vi "PanelPrincipal.vi"() -> ()   [LabVIEW 2020]
panel:
  out "Waveform Chart":dynamicdata(graph)
  out "V2":bool
  out "Motor2":bool
  out "Motor1":bool
  out "V1":bool
  in  "stop":bool caption="Parada"
  out "Multi-Segment Pipe 7":bool(c317)
  out "Tanque 2":dbl(slide) scale=0.0..100.0 scale format="%#.2g"
  out "Multi-Segment Pipe 4":bool(c317)
  out "Flujo":dbl
  out "Multi-Segment Pipe 6":bool(c317)
  out "Multi-Segment Pipe 5":bool(c317)
  out "Multi-Segment Pipe 3":bool(c317)
  out "Multi-Segment Pipe 2":bool(c317)
  out "Tanque 1":dbl(slide) scale=0.0..100.0 scale format="%#.2g"
  out "Multi-Segment Pipe":bool(c317)
  out "Thermometer":dbl(slide) caption="Termómetro" scale=0.0..100.0
  # "M2"
  # "M1"
  # "Nivel"
  # "V2"
  # "V1"
  # "D1"
  # "D2"
  # "G2"
  # "G1"
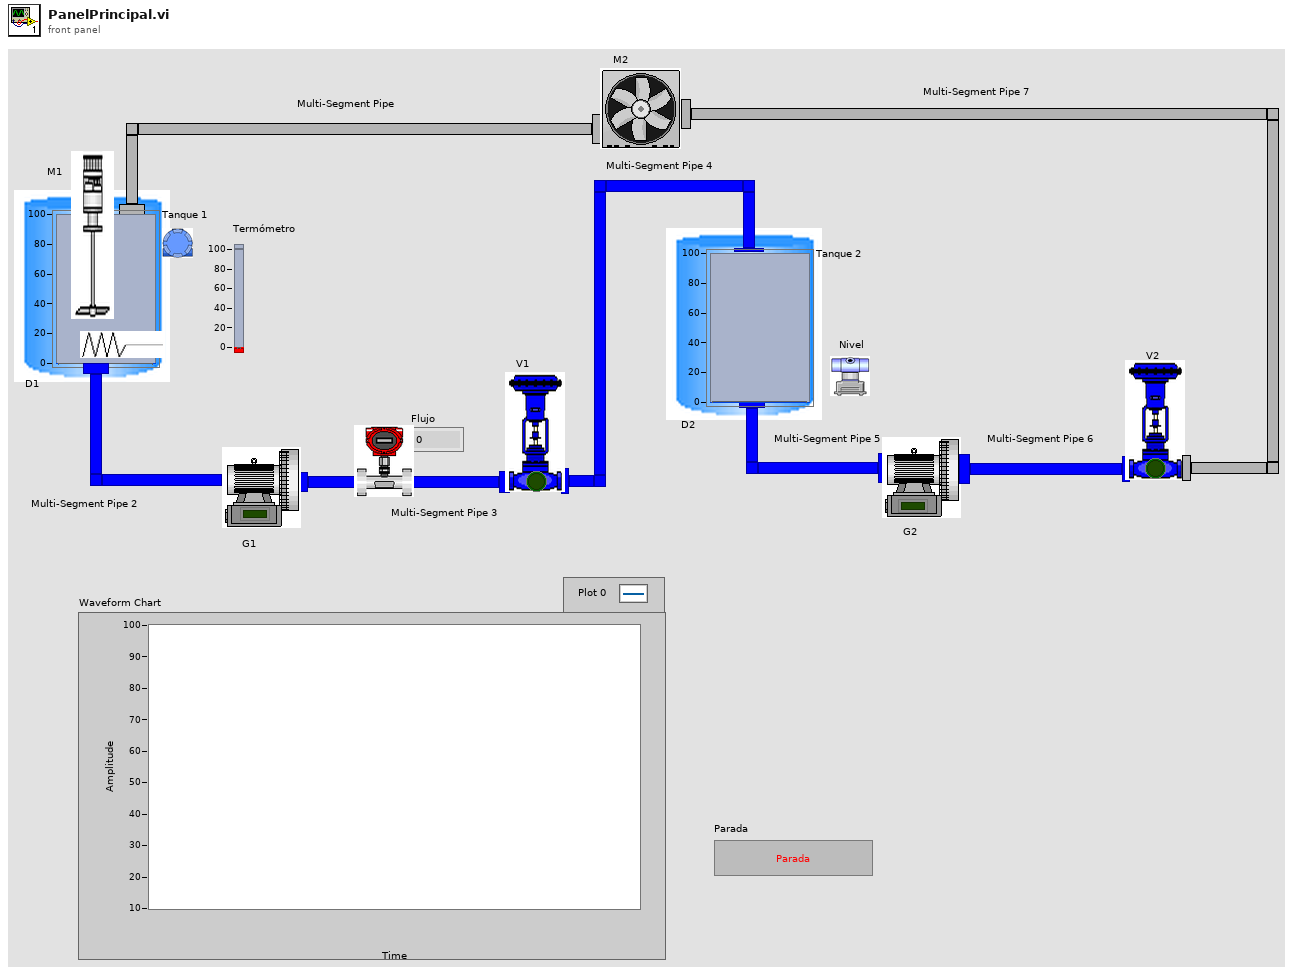
[diagram p1: front panel]
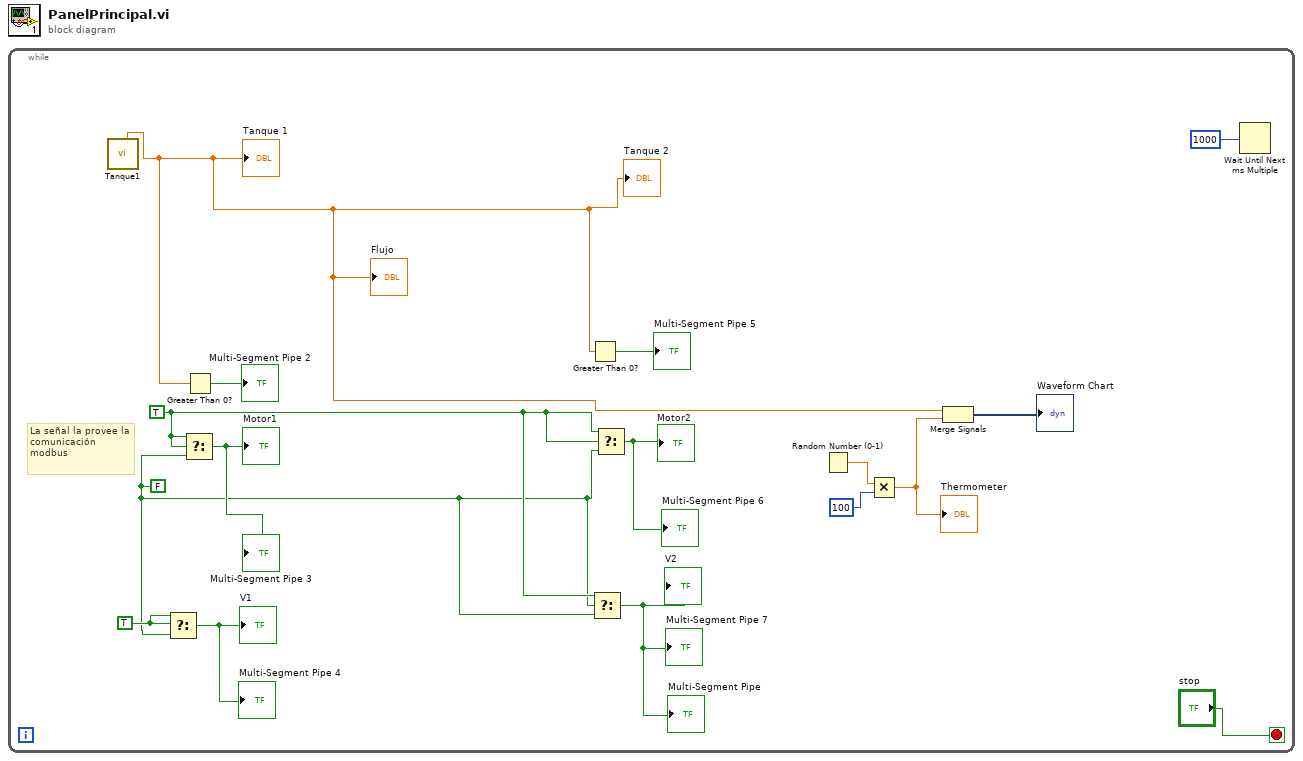
[diagram p0: block diagram]
diagram:
  n1 = while {
    stop <- "stop" stop-if-true
    w12 = TRUE
    w7 = FALSE
    w8 = TRUE
    # "La señal la provee la comunicación modbus"
    n2 = call "Tanque1.vi"() -> ("Numeric"=w5:dbl)  [unwired: 11 in]
    "Tanque 1" <- w5
    "Tanque 2" <- w5
    "Flujo" <- w5
    n3 = Select(t=w12, s=w12, f=w7) -> (s? t:f=→"Multi-Segment Pipe 4" →"V1":bool)
    n4 = Select(t=w8, s=w8, f=w7) -> (s? t:f=→"Multi-Segment Pipe 3" →"Motor1":bool)
    n5 = Greater Than 0?(x=w5) -> (x > 0?=→"Multi-Segment Pipe 2":bool)
    n6 = Greater Than 0?(x=w5) -> (x > 0?=→"Multi-Segment Pipe 5":bool)
    n7 = Select(t=w8, s=w7, f=w7) -> (s? t:f=→"Multi-Segment Pipe" →"Multi-Segment Pipe 7" →"V2":bool)
    n8 = Select(t=w8, s=w8, f=w7) -> (s? t:f=→"Multi-Segment Pipe 6" →"Motor2":bool)
    n9 = Random Number (0-1)() -> (number: 0 to 1=w4:dbl)
    n10 = Multiply(x=w4, y=100) -> (x*y=w2:dbl)
    "Thermometer" <- w2
    n11 = Merge Signals(w5, w2) -> (→"Waveform Chart":dynamicdata)
    n12 = Wait Until Next ms Multiple(millisecond multiple=1000) -> ()  [unwired: 1 out]
  }
